vi "GetGitHash.vi"(8 "error in (no error)":errorcluster, 11 "Path":path) -> (0 "error out":errorcluster, 3 "Hash":string)   [LabVIEW 2012]
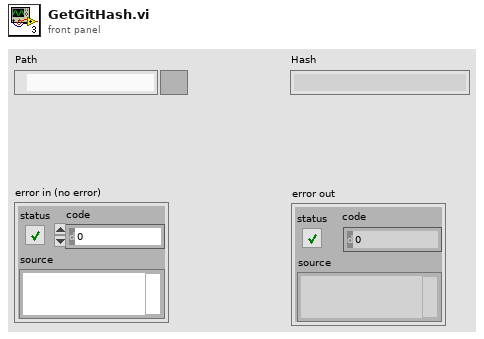
[diagram p1: front panel]
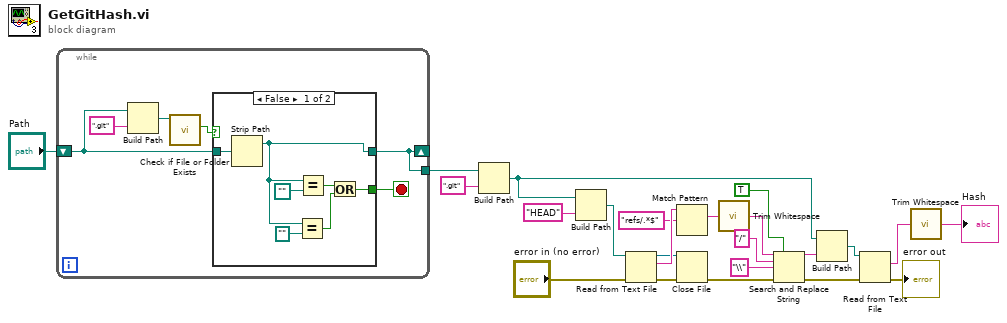
[diagram p0: block diagram]
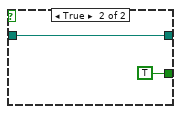
[diagram p2: hidden frame]
diagram:
  n1 = while {
    shift-right: [w25] -> _
    shift-left: "Path" -> [w26]
    tunnel: [w25] -> w1
    stop <- w24 stop-if-true
    n2 = Build Path(base path=w26, name or relative path=".git") -> (appended path=w28:path)
    n3 = call <vilib>:"Check if File or Folder Exists.vi"("path"=w28) -> ("file or folder exists?"=w27:bool)  [unwired: 8 in, 2 out]
    n4 = case shown="False" w27 {
      tunnel: [w34 w37] -> w25
      tunnel: w26 -> [w36 w37]
      tunnel: [w30 TRUE] -> w24
      frame False {
        n5 = Strip Path(path=w36) -> (stripped path=w34:path)  [unwired: 1 out]
        n6 = Equal?(x=w34, y=path "") -> (x = y?=w31:bool)
        n7 = Equal?(x=w34, y=path "") -> (x = y?=w32:bool)
        n8 = Or(x=w32, y=w31) -> (x .or. y?=w30:bool)
      }
      frame True {
      }
    }
  }
  n9 = Build Path(base path=w1, name or relative path=".git") -> (appended path=w17:path)
  n10 = Build Path(base path=w17, name or relative path="HEAD") -> (appended path=w21:path)
  n11 = Read from Text File(file (use dialog)=w21, error in="error in (no error)") -> (refnum out=w15:refnum<file>, text=w19:string, error out=w16:errorcluster)  [unwired: 2 in, 1 out]
  n12 = Match Pattern(string=w19, regular expression="refs/.*$") -> (match substring=w10:string)  [unwired: 1 in, 3 out]
  n13 = Close File(refnum=w15, error in=w16) -> (error out=w6:errorcluster)  [unwired: 1 out]
  n14 = call <vilib>:"Trim Whitespace.vi"("string"=w10) -> ("trimmed string"=w9:string)  [unwired: 1 in]
  n15 = Search and Replace String(replace all?=TRUE, input string=w9, search string="/", replace string="\\", error in=w6) -> (result string=w11:string, error out=w5:errorcluster)  [unwired: 3 in, 2 out]
  n16 = Build Path(base path=w17, name or relative path=w11) -> (appended path=w8:path)
  n17 = Read from Text File(file (use dialog)=w8, error in=w5) -> (text=w4:string, error out=→"error out":errorcluster)  [unwired: 2 in, 2 out]
  n18 = call <vilib>:"Trim Whitespace.vi"("string"=w4) -> ("trimmed string"=→"Hash":string)  [unwired: 1 in]
